vi "查找元素.vi"(6 "error in (no error)":errorcluster caption="错误输入（无错误）", 8 "offset (0)":i32 caption="偏移量(0)", 11 "XML String In":string caption="XML字符串输入") -> (0 "offset past match":i32 caption="匹配后偏移量", 1 "after  tag":string caption="标识符之后", 2 "tag":string caption="标识符", 3 "before tag":string caption="标识符之前", 4 "error out":errorcluster caption="错误输出", 5 "element name":string caption="元素名", 7 "节点名":string)   [LabVIEW 2017]
uses:
  <vilib>/regexp/Match Regular Expression.xnode
panel:
  # "<编号 id=“01”>测试<\\编号>"
  # "<编号ID 序号=\"1\">200</编号ID>"
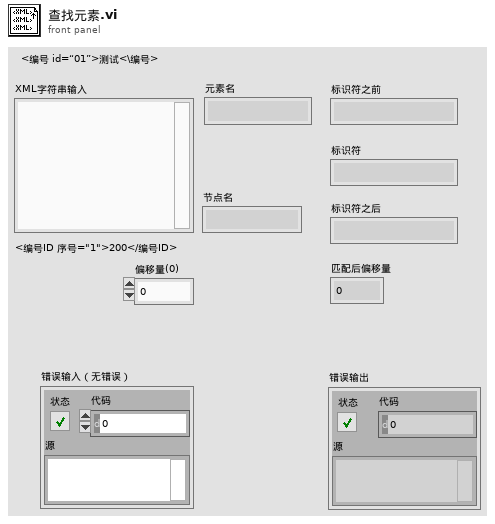
[diagram p1: front panel]
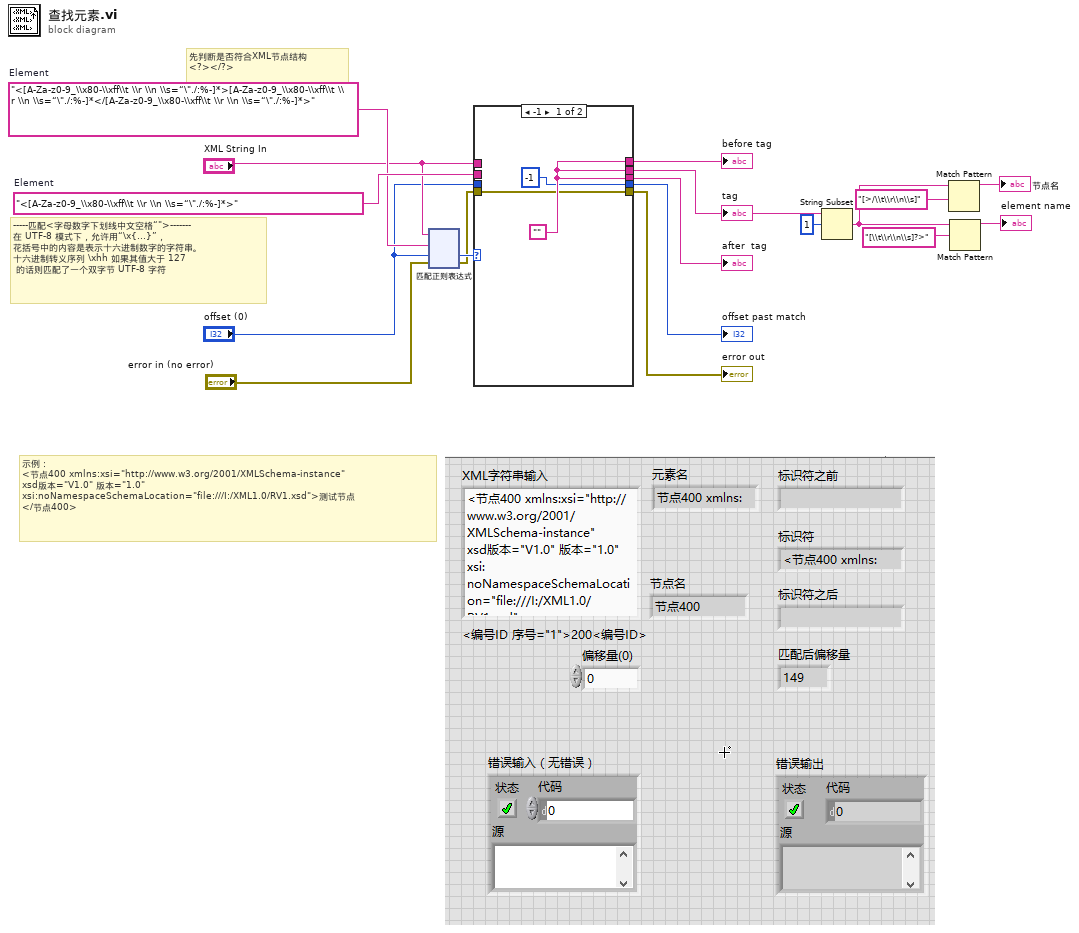
[diagram p0: block diagram]
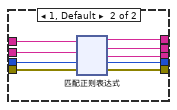
[diagram p2: hidden frame]
diagram:
  w5 = "<[A-Za-z0-9_\\x80-\\xff\\t \\r \\n \\s=“\"./:%-]*>[A-Za-z0-9_\\x80-\\xff\\t \\r \\n \\s=“\"./:%-]*</[A-Za-z0-9_\\x80-\\xff\\t \\r \\n \\s=“\"./:%-]*>"  # Element
  w14 = "<[A-Za-z0-9_\\x80-\\xff\\t \\r \\n \\s=“\"./:%-]*>"  # Element
  # "先判断是否符合XML节点结构\n<?></?>"
  # "示例：\n<节点400 xmlns:xsi=\"http://www.w3.org/2001/XMLSchema-instance\" \nxsd版本=\"V1.0\" 版本=\"1.0\" \nxsi:noNamespaceSchemaLocation=\"file:///I:/XML1.0/RV1.xsd\">测试节点\n</节点400>"
  # "-----匹配<字母数字下划线中文空格“\">-------\n在 UTF-8 模式下，允许用“\\x{...}”，\n花括号中的内容是表示十六进制数字的字符串。\n十六进制转义序列 \\xhh 如果其值大于 127\n 的话则匹配了一个双字节 UTF-8 字符"
  n1 = xnode "匹配正则表达式"("输入字符串"="XML String In", "正则表达式"=w5, "偏移量(0)"="offset (0)", "错误输入"="error in (no error)") -> ("匹配后偏移量"=w6:i32, "错误输出"=w2:errorcluster)  [unwired: 2 in, 3 out]
  n2 = case shown="-1" w6 {
    tunnel: [w21 w30] -> w18
    tunnel: [w21 w29] -> w17
    tunnel: "offset (0)" -> [_ w28]
    tunnel: w14 -> [_ w27]
    tunnel: "XML String In" -> [_ w26]
    tunnel: [-1 ("匹配后偏移量") w25] -> w13
    tunnel: w2 -> [w19 w24]
    tunnel: [w19 w23] -> w12
    tunnel: [w21 w22] -> w10
    frame -1 {
      w21 = ""
    }
    frame 1, Default {
      n3 = xnode "匹配正则表达式"("输入字符串"=w26, "正则表达式"=w27, "偏移量(0)"=w28, "错误输入"=w24) -> ("匹配之前"=w30:string, "所有匹配"=w22:string, "匹配之后"=w29:string, "匹配后偏移量"=w25:i32, "错误输出"=w23:errorcluster)  [unwired: 2 in]
    }
  }
  "offset past match" <- w13
  "before tag" <- w18
  "tag" <- w10
  "after  tag" <- w17
  "error out" <- w12
  n4 = String Subset(string=w10, offset (0)=1) -> (substring=w7:string)  [unwired: 1 in]
  n5 = Match Pattern(string=w7, regular expression="[>/\\t\\r\\n\\s]") -> (before substring=→"节点名":string)  [unwired: 1 in, 3 out]
  n6 = Match Pattern(string=w7, regular expression="[\\t\\r\\n\\s]?>") -> (before substring=→"element name":string)  [unwired: 1 in, 3 out]
